vi "Wait for Return FIFO.vi"(6 "infinite timeout? (F)":bool, 8 "error in (no error)":errorcluster, 9 "timeout (0 ms)":i32 format="%d ms", 11 "Transfer Group Bundle in":refnum<class "Scheduler Transfer Group Bundle.lvclass">) -> (0 "error out":errorcluster, 2 "iteration valid":bool, 3 "Transfer Group Bundle out":refnum<class "Scheduler Transfer Group Bundle.lvclass">)   [LabVIEW 2017, in "Scheduler Transfer Group Bundle.lvclass"]
uses:
  Scheduler/Scheduler Transfer Group Bundle.lvclass
  Timing.lvclass
  Transfer Group Timing.lvclass
  C:/Git/DSF/Data Sharing Framework/Source/Core/Engine/Classes/Timing/Timing.lvclass
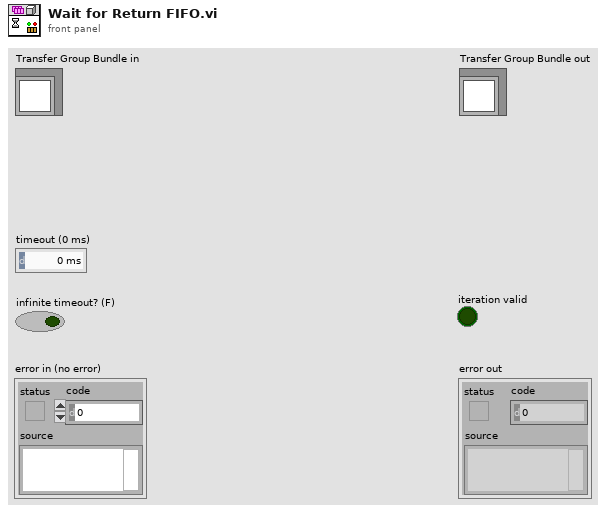
[diagram p1: front panel]
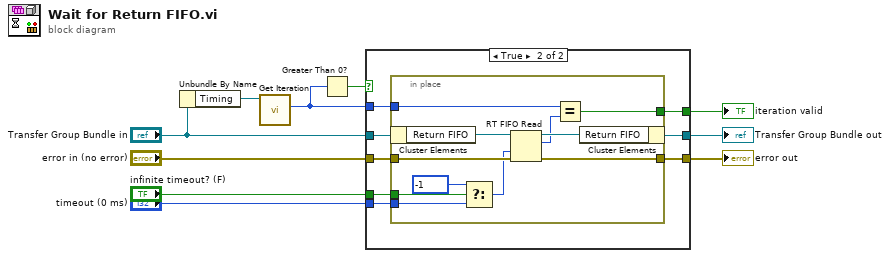
[diagram p0: block diagram]
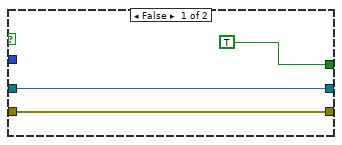
[diagram p2: hidden frame]
diagram:
  n1 = Unbundle By Name("Transfer Group Bundle in") -> ("Timing"=w2:refnum<class "Transfer Group Timing.lvclass">)
  n2 = call "Get Iteration.vi"("Timing in"=w2) -> ("Iteration"=w6:u64)  [unwired: 9 in, 1 out]
  n3 = Greater Than 0?(x=w6) -> (x > 0?=w7:bool)
  n4 = case shown="True" w7 {
    tunnel: "error in (no error)" -> [w12 w21]
    tunnel: [w12 w20] -> w9
    tunnel: "Transfer Group Bundle in" -> [w13 w15]
    tunnel: [w13 w14] -> w8
    tunnel: w6 -> [_ w19]
    tunnel: [TRUE w18] -> w5
    tunnel: "infinite timeout? (F)" -> [_ w17]
    tunnel: "timeout (0 ms)" -> [_ w16]
    frame False {
    }
    frame True {
      n5 = in-place {
        in-place-border: w21 -> [w31]
        in-place-border: [w30] -> w20
        in-place-border: w19 -> [w28]
        in-place-border: [w27] -> w18
        in-place-border: w17 -> [w26]
        in-place-border: w16 -> [w25]
        n6 = in-place-cluster #1(w15) -> ("Return FIFO"=w24:refnum<k33>)
        n7 = Select(t=-1, s=w26, f=w25) -> (s? t:f=w29:i32)
        n8 = RT FIFO Read(0:w24, 2:w29, 3:w31) -> (8:w23:refnum<k33>, 9:w22:u64, 11:w30:errorcluster)  [unwired: 1 in, 2 out]
        n9 = Equal?(x=w28, y=w22) -> (x = y?=w27:bool)
        n10 = in-place-cluster #1("Return FIFO"=w23) -> (w14:refnum<class "Scheduler Transfer Group Bundle.lvclass">)
      }
    }
  }
  "error out" <- w9
  "Transfer Group Bundle out" <- w8
  "iteration valid" <- w5
